vi "CS-4 Get Limits.vi"(6 "error in (no error)":errorcluster, 9 "VISA session":refnum<visa-resource-name>) -> (0 "error out":errorcluster, 1 "lower sweep limit":dbl format="%.2f", 2 "upper sweep limit":dbl format="%.2f", 3 "dup VISA session":refnum<visa-resource-name>, 4 "voltage limit":dbl format="%.2f")   [LabVIEW 2016]
doc: "CS-4 Get Limits.vi will return the upper and lower sweep limits and voltage limit."
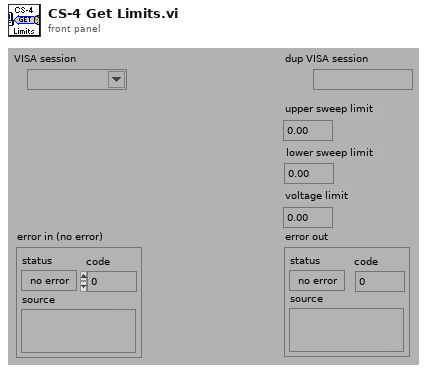
[diagram p1: front panel]
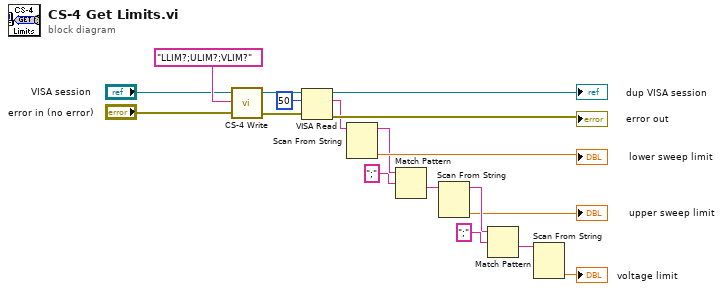
[diagram p0: block diagram]
diagram:
  n1 = call "CS-4 Write.vi"("error in (no error)"="error in (no error)", "write buffer (\"\")"="LLIM?;ULIM?;VLIM?", "VISA session"="VISA session") -> ("error out"=w10:errorcluster, "dup VISA session"=w11:refnum<visa-resource-name>)  [unwired: 1 out]
  n2 = VISA Read(VISA resource name=w11, byte count=u32 50 ("byte count (0)"), error in (no error)=w10) -> (VISA resource name out=→"dup VISA session":refnum<visa-resource-name>, read buffer=w14:string, error out=→"error out":errorcluster)  [unwired: 1 out]
  n3 = Scan From String(input string=w14) -> (remaining string=w8:string, output 1=→"lower sweep limit":dbl)  [unwired: 4 in, 2 out]
  n4 = Match Pattern(string=w8, regular expression=";") -> (after substring=w4:string)  [unwired: 1 in, 3 out]
  n5 = Scan From String(input string=w4) -> (remaining string=w5:string, output 1=→"upper sweep limit":dbl)  [unwired: 4 in, 2 out]
  n6 = Match Pattern(string=w5, regular expression=";") -> (after substring=w2:string)  [unwired: 1 in, 3 out]
  n7 = Scan From String(input string=w2) -> (output 1=→"voltage limit":dbl)  [unwired: 4 in, 3 out]
